vi "pl1000GetSingle.vi"(8 "error in (no error)":errorcluster, 10 "channel":i32=1, 11 "pl1000 handle":i16) -> (0 "error out":errorcluster, 2 "value":u16, 3 "pl1000 handle out":i16)   [LabVIEW 2016, in "pl1000.lvlib"]
doc: "This function returns a single sample value from the specified input channel.\n\nchannel: which channel to sample"
uses:
  pl1000.lvlib
  pl1000.dll
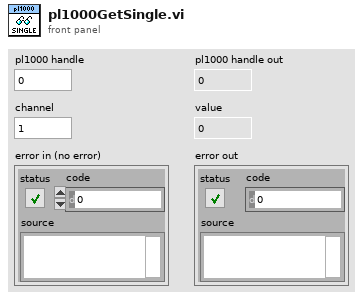
[diagram p1: front panel]
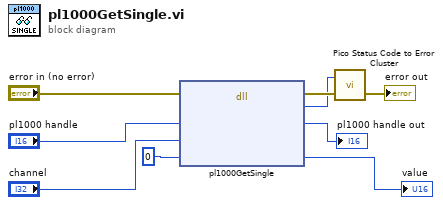
[diagram p0: block diagram]
diagram:
  n1 = dll-call lib="pl1000.dll" fn="pl1000GetSingle"(error in="error in (no error)", "handle"="pl1000 handle", "channel"="channel", "value"=u16 0) -> (error out=w7:errorcluster, "status"=w6:u32, "handle"=→"pl1000 handle out":i16, "value"=→"value":u16)  [unwired: 3 in, 1 out]
  n2 = call "Pico Status Code to Error Cluster.vi"("error in"=w7, "PICO_STATUS"=w6) -> ("error out"=→"error out":errorcluster)  [unwired: 1 in]
